vi "Write Test Results to Front Panel.vi"(8 "error in (no error)":errorcluster, 10 "Current State":T1) -> (0 "error out":errorcluster)   [LabVIEW 2014]
uses:
  Controls/States.ctl
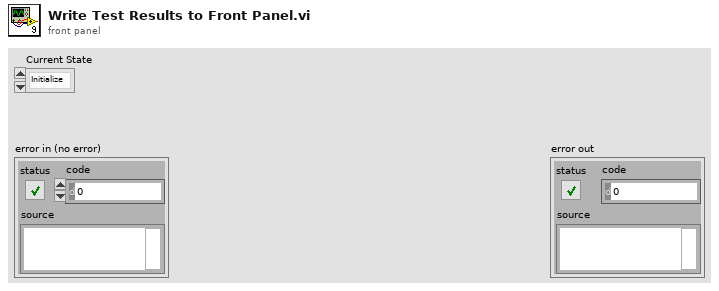
[diagram p1: front panel]
types:
  T1 = typedef "States.ctl" = enum16{"Initialize", "Wait for User Input", "Check User Input", "Insert Open VI", "Run Open VI", "Straight Line", "Home", "Limit", "Generate Report", "Finalize", "Terminate"}
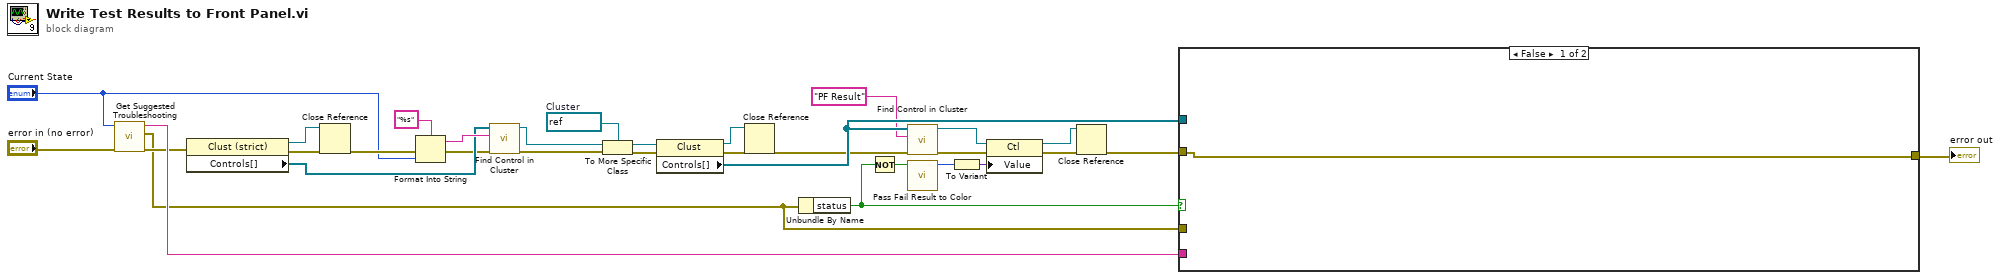
[diagram p0: block diagram]
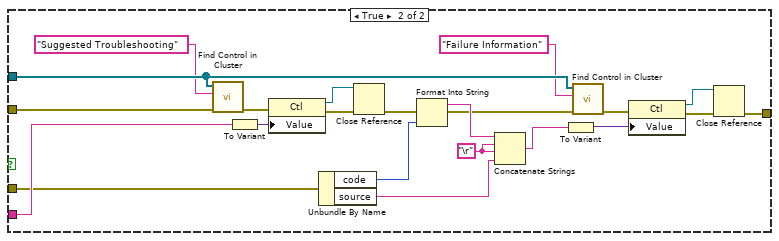
[diagram p2: hidden frame]
diagram:
  w10 = refnum<vi> refnum  # Cluster
  n1 = call "Get Suggested Troubleshooting.vi"("error in (no error)"="error in (no error)", "Current State"="Current State") -> ("error out"=w5:errorcluster, "Test Error"=w2:errorcluster, "Suggested Troubleshooting"=w6:string)  [unwired: 7 in]
  n2 = property class="Clust (strict)"(error in=w5) -> (reference out=w20:refnum<vi>, error out=w18:errorcluster, "Controls[]"=w22:refnum<vi>[])  [unwired: 1 in]
  n3 = Close Reference(reference=w20, error in (no error)=w18) -> (error out=w19:errorcluster)
  n4 = Format Into String(format string="%s", error in=w19, "Current State") -> (resulting string=w23:string, error out=w21:errorcluster)  [unwired: 1 in]
  n5 = call "Find Control in Cluster.vi"("error in (no error)"=w21, "String"=w23, "Controls[]"=w22) -> ("error out"=w25:errorcluster, "Control out"=w24:refnum<vi>)  [unwired: 7 in]
  n6 = To More Specific Class(target class=w10, reference=w24, error in=w25) -> (specific class reference=w11:refnum<vi>, error out=w12:errorcluster)
  n7 = property class="Clust"(reference=w11, error in=w12) -> (reference out=w27:refnum<vi>, error out=w26:errorcluster, "Controls[]"=w32:refnum<vi>[])
  n8 = Close Reference(reference=w27, error in (no error)=w26) -> (error out=w28:errorcluster)
  n9 = Unbundle By Name(w2) -> ("status"=w3:bool)
  n10 = Not(x=w3) -> (.not. x?=w4:bool)
  n11 = call "Find Control in Cluster.vi"("error in (no error)"=w28, "String"="PF Result", "Controls[]"=w32) -> ("error out"=w14:errorcluster, "Control out"=w15:refnum<vi>)  [unwired: 7 in]
  n12 = call "Pass Fail Result to Color.vi"("Pass?"=w4) -> ("Color Value"=w17:u32)  [unwired: 10 in]
  n13 = To Variant(anything=w17) -> (Variant=w16:variant)
  n14 = property class="Ctl"(reference=w15, error in=w14, "Value"=w16) -> (reference out=w30:refnum<vi>, error out=w29:errorcluster)
  n15 = Close Reference(reference=w30, error in (no error)=w29) -> (error out=w31:errorcluster)
  n16 = case shown="False" w3 {
    tunnel: w32 -> [_ w55]
    tunnel: w31 -> [w33 w48]
    tunnel: [w33 w43] -> w7
    tunnel: w6 -> [_ w42]
    tunnel: w2 -> [_ w41]
    frame False {
    }
    frame True {
      w36 = "\r"
      n17 = call "Find Control in Cluster.vi"("error in (no error)"=w48, "String"="Suggested Troubleshooting", "Controls[]"=w55) -> ("error out"=w44:errorcluster)  [unwired: 7 in, 1 out]
      n18 = To Variant(anything=w42) -> (Variant=w49:variant)
      n19 = property class="Ctl"(error in=w44, "Value"=w49) -> (reference out=w46:refnum<vi>, error out=w47:errorcluster)  [unwired: 1 in]
      n20 = Unbundle By Name(w41) -> ("code"=w40:i32, "source"=w37:string)
      n21 = Close Reference(reference=w46, error in (no error)=w47) -> (error out=w39:errorcluster)
      n22 = Format Into String(error in=w39, w40) -> (resulting string=w38:string, error out=w34:errorcluster)  [unwired: 2 in]
      n23 = Concatenate Strings(w38, w36, w36, w37) -> (w35:string)
      n24 = To Variant(anything=w35) -> (Variant=w50:variant)
      n25 = call "Find Control in Cluster.vi"("error in (no error)"=w34, "String"="Failure Information", "Controls[]"=w55) -> ("error out"=w53:errorcluster)  [unwired: 7 in, 1 out]
      n26 = property class="Ctl"(error in=w53, "Value"=w50) -> (reference out=w52:refnum<vi>, error out=w51:errorcluster)  [unwired: 1 in]
      n27 = Close Reference(reference=w52, error in (no error)=w51) -> (error out=w43:errorcluster)
    }
  }
  "error out" <- w7
